vi "Configure Track Write Operation.vi"(4 "Specify a Channel":T2, 5 "Enable":bool, 6 "Track Name":string, 7 "Error In":errorcluster, 8 "Write Position":i64, 9 "Track Data":T1, 10 "Track (File) Reference In":refnum<k34>) -> (0 "Error Out":errorcluster, 3 "Track (File) Reference Out":refnum<k34>)   [LabVIEW 2014]
doc: "Performs some configuration operation that must be done before a TDMS write VI can be called. The configuration is based on the Track file format that was chosen."
uses:
  Controls/Specifiy a Channel.ctl
  Controls/Audio In.ctl
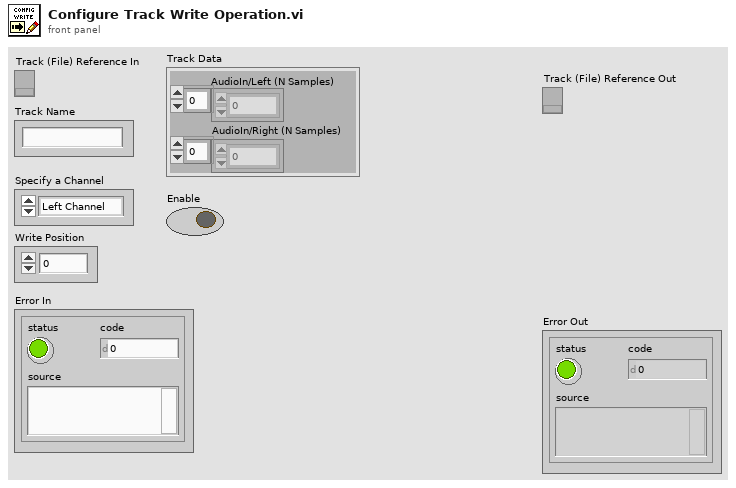
[diagram p1: front panel]
types:
  T1 = typedef "Audio In.ctl" = cluster{"AudioIn/Left (N Samples)":i16[], "AudioIn/Right (N Samples)":i16[]}
  T2 = typedef "Specifiy a Channel.ctl" = enum16{"Left Channel", "Right Channel", "Both Channels"}
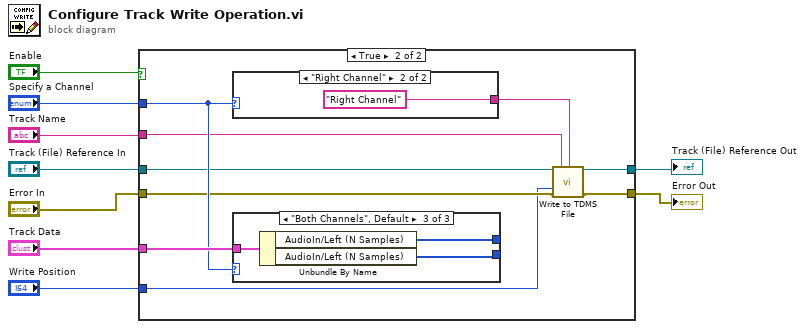
[diagram p0: block diagram]
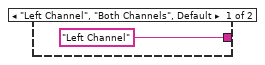
[diagram p3: hidden frame]
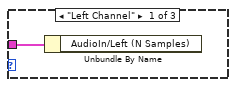
[diagram p4: hidden frame]
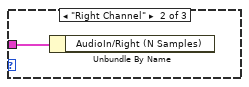
[diagram p5: hidden frame]
diagram:
  n1 = case shown="True" "Enable" {
    tunnel: "Error In" -> [w11 w15]
    tunnel: "Write Position" -> [_ w14]
    tunnel: [w11 w13] -> w9
    tunnel: "Track Data" -> [_ w20]
    tunnel: "Track Name" -> [_ w18]
    tunnel: "Track (File) Reference In" -> [w10 w16]
    tunnel: "Specify a Channel" -> [_ w19]
    tunnel: [w10 w12] -> w1
    frame False {
    }
    frame True {
      n2 = case shown="\"Right Channel\"" w19 {
        tunnel: ["Left Channel" "Right Channel"] -> w17
        frame "Left Channel", "Both Channels", Default {
        }
        frame "Right Channel" {
        }
      }
      n3 = case shown="\"Both Channels\", Default" w19 {
        tunnel: w20 -> [w24 w26 w29]
        tunnel: [_ _ w28] -> _
        tunnel: [_ _ w27] -> _
        frame "Left Channel" {
          n4 = Unbundle By Name(w24) -> ("AudioIn/Left (N Samples)"=w23:i16[])
        }
        frame "Right Channel" {
          n5 = Unbundle By Name(w26) -> ("AudioIn/Right (N Samples)"=w25:i16[])
        }
        frame "Both Channels", Default {
          n6 = Unbundle By Name(w29) -> ("AudioIn/Left (N Samples)"=w28:i16[], "AudioIn/Left (N Samples)"=w27:i16[])
        }
      }
      n7 = call "Write to TDMS File.vi"("TDMS Reference In"=w16, "Track Name"=w18, "Channel Name"=w17, "Write Position"=w14, "Error In"=w15) -> ("TDMS Reference Out"=w12:refnum<k34>, "Error Out"=w13:errorcluster)  [unwired: 9 in]
    }
  }
  "Error Out" <- w9
  "Track (File) Reference Out" <- w1
